vi "BuildVI.vi"(8 "error in (no error)":errorcluster, 10 "Name":string, 11 "CreateClass In":refnum<class "CreateClass.lvclass">) -> (0 "error out":errorcluster, 3 "CreateClass Out":refnum<class "CreateClass.lvclass">)   [LabVIEW 2020, in "Mermaid.lvlib" / "CreateClass.lvclass"]
uses:
  CreateClass.lvclass
  CreateClass.lvclass/CreateClass.ctl
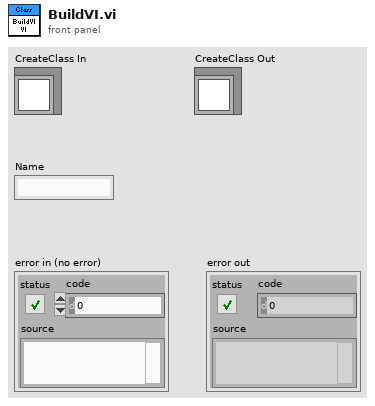
[diagram p1: front panel]
types:
  T1 = enum32{"invalid VI type", "Standard VI", "Control VI", "Global VI", "Polymorphic VI", "Configuration VI", "SubSystem", "Facade VI", "Method VI", "Statechart Diagram VI"}
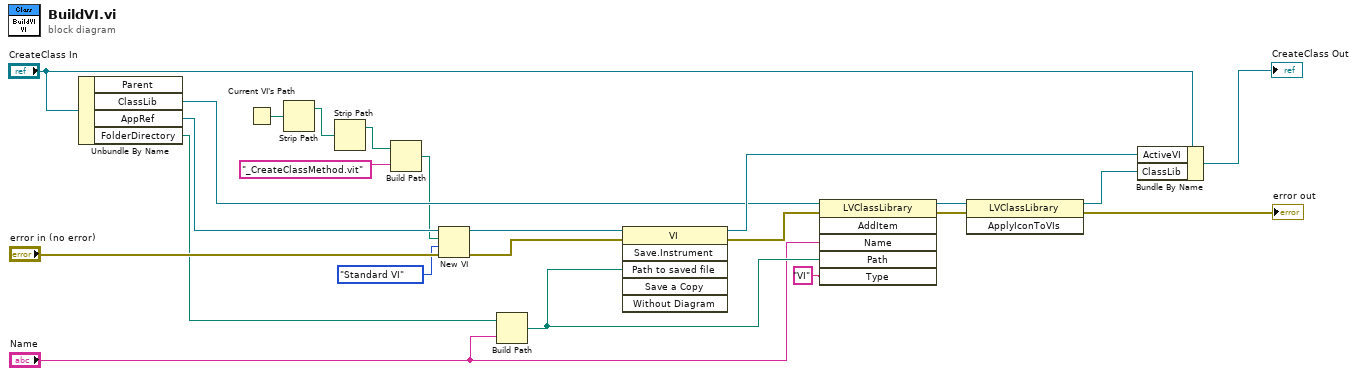
[diagram p0: block diagram]
diagram:
  n1 = Unbundle By Name("CreateClass In") -> ("ClassLib"=w20:refnum<vi>, "AppRef"=w19:refnum<vi>, "FolderDirectory"=w8:path)  [unwired: 1 out]
  n2 = Current VI's Path() -> (path=w4:path)
  n3 = Strip Path(path=w4) -> (stripped path=w3:path)  [unwired: 1 out]
  n4 = Strip Path(path=w3) -> (stripped path=w2:path)  [unwired: 1 out]
  n5 = Build Path(base path=w2, name or relative path="_CreateClassMethod.vit" ("Name")) -> (appended path=w15:path)
  n6 = New VI(8:"error in (no error)", 9:T1."Standard VI" ("vi type (standard vi)"), 10:w15, 11:w19) -> (0:w10:errorcluster, 3:w9:refnum<vi>)  [unwired: 3 in]
  n7 = Build Path(base path=w8, name or relative path="Name") -> (appended path=w12:path)
  n8 = invoke class="VI" method="Save.Instrument"(reference=w9, error in=w10, "Path to saved file"=w12) -> (reference out=w21:refnum<vi>, error out=w11:errorcluster)  [unwired: 3 in, 4 out]
  n9 = invoke class="LVClassLibrary" method="AddItem"(reference=w20, error in=w11, "Name"="Name", "Path"=w12, "Type"="VI") -> (reference out=w16:refnum<vi>, error out=w17:errorcluster)  [unwired: 1 in, 4 out]
  n10 = invoke class="LVClassLibrary" method="ApplyIconToVIs"(reference=w16, error in=w17) -> (reference out=w23:refnum<vi>, error out=→"error out":errorcluster)  [unwired: 1 in, 1 out]
  n11 = Bundle By Name(cluster="CreateClass In", "ActiveVI"=w21, "ClassLib"=w23) -> (→"CreateClass Out":refnum<class "CreateClass.lvclass">)
